vi "H_ofAllPoints.vi"(10 "Temperature Sensors":T2, 11 "Pressure Sensors in":T1) -> (3 "H's":dbl[](array[numeric]))   [LabVIEW 2017]
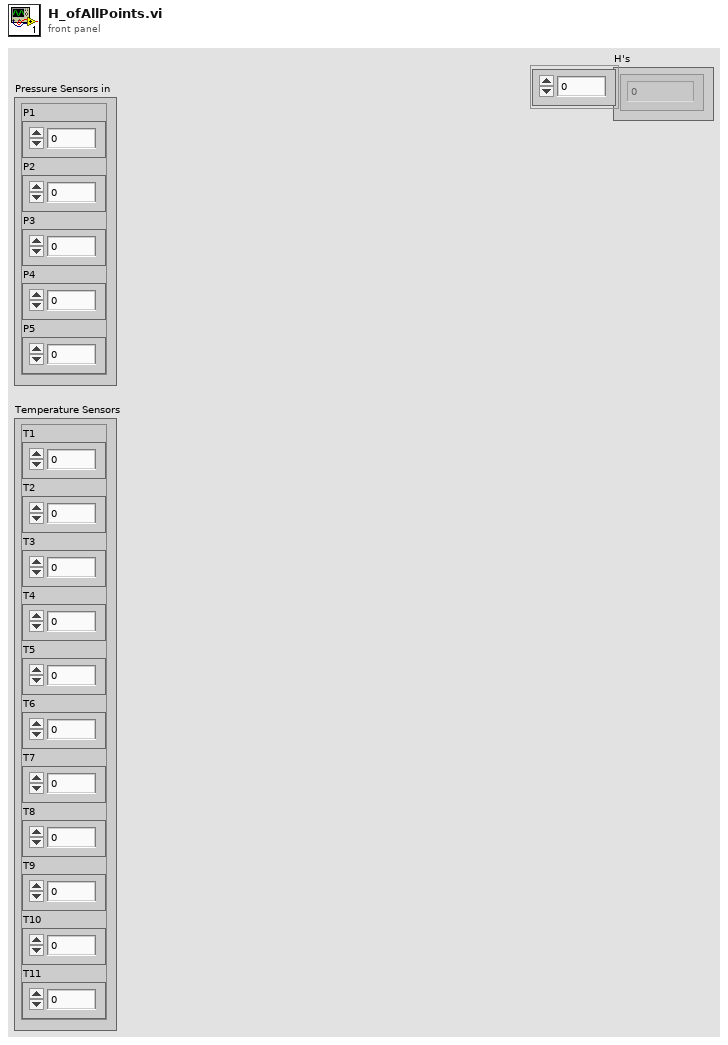
[diagram p1: front panel]
types:
  T1 = cluster{"P1":dbl, "P2":dbl, "P3":dbl, "P4":dbl, "P5":dbl}
  T2 = cluster{"T1":dbl, "T2":dbl, "T3":dbl, "T4":dbl, "T5":dbl, "T6":dbl, "T7":dbl, "T8":dbl, "T9":dbl, "T10":dbl, "T11":dbl}
  T3 = cluster{"S":dbl, "H":dbl, "V":dbl, "T":dbl, "P":dbl, "Status":enum16{"Sub Cooled", "Saturation", "Super Heated"}, "S 2":dbl, "H 2":dbl, "V 2":dbl, "T No":enum16{"0", "1", "2", "3", "4"}, "quality":dbl}
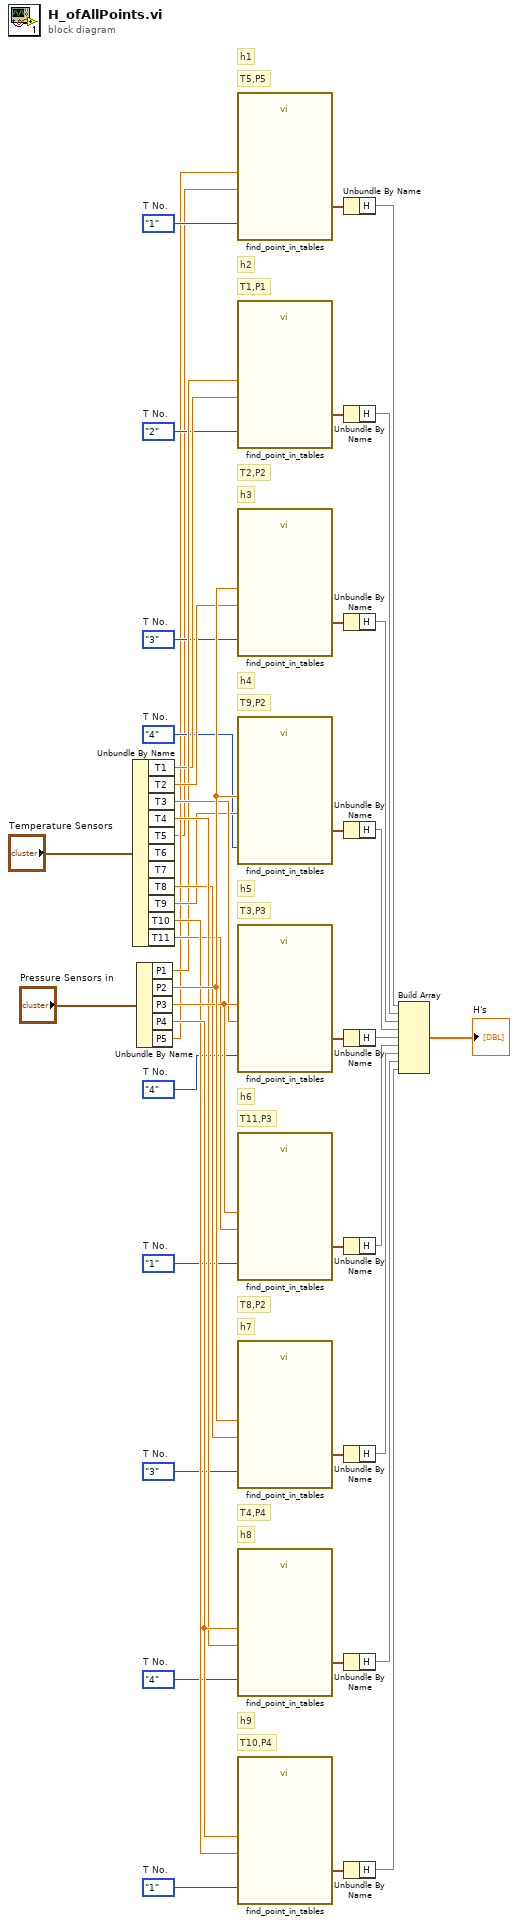
[diagram p0: block diagram]
diagram:
  w20 = enum16{"0", "1", "2", "3", "4"}."1"  # T No.
  w19 = enum16{"0", "1", "2", "3", "4"}."4"  # T No.
  w16 = enum16{"0", "1", "2", "3", "4"}."3"  # T No.
  w15 = enum16{"0", "1", "2", "3", "4"}."1"  # T No.
  w12 = enum16{"0", "1", "2", "3", "4"}."4"  # T No.
  w11 = enum16{"0", "1", "2", "3", "4"}."4"  # T No.
  w8 = enum16{"0", "1", "2", "3", "4"}."3"  # T No.
  w7 = enum16{"0", "1", "2", "3", "4"}."2"  # T No.
  w4 = enum16{"0", "1", "2", "3", "4"}."1"  # T No.
  # "T10,P4"
  # "T4,P4"
  # "T8,P2"
  # "T11,P3"
  # "T3,P3"
  # "T9,P2"
  # "T2,P2"
  # "T1,P1"
  # "T5,P5"
  # "h9"
  # "h8"
  # "h7"
  # "h6"
  # "h5"
  # "h4"
  # "h3"
  # "h2"
  # "h1"
  n1 = Unbundle By Name("Temperature Sensors") -> ("T1"=w22:dbl, "T2"=w24:dbl, "T3"=w26:dbl, "T4"=w29:dbl, "T5"=w2:dbl, "T8"=w28:dbl, "T9"=w25:dbl, "T10"=w30:dbl, "T11"=w27:dbl)  [unwired: 2 out]
  n2 = Unbundle By Name("Pressure Sensors in") -> ("P1"=w23:dbl, "P2"=w32:dbl, "P3"=w31:dbl, "P4"=w33:dbl, "P5"=w3:dbl)
  n3 = call "find_point_in_tables.vi"("T No."=w4, "T Search"=w2, "P Search"=w3) -> ("Point"=w5:T3)  [unwired: 7 in]
  n4 = call "find_point_in_tables.vi"("T No."=w7, "T Search"=w22, "P Search"=w23) -> ("Point"=w6:T3)  [unwired: 7 in]
  n5 = call "find_point_in_tables.vi"("T No."=w8, "T Search"=w24, "P Search"=w32) -> ("Point"=w9:T3)  [unwired: 7 in]
  n6 = call "find_point_in_tables.vi"("T No."=w11, "T Search"=w25, "P Search"=w32) -> ("Point"=w10:T3)  [unwired: 7 in]
  n7 = call "find_point_in_tables.vi"("T No."=w12, "T Search"=w26, "P Search"=w31) -> ("Point"=w13:T3)  [unwired: 7 in]
  n8 = call "find_point_in_tables.vi"("T No."=w15, "T Search"=w27, "P Search"=w31) -> ("Point"=w14:T3)  [unwired: 7 in]
  n9 = call "find_point_in_tables.vi"("T No."=w16, "T Search"=w28, "P Search"=w32) -> ("Point"=w17:T3)  [unwired: 7 in]
  n10 = call "find_point_in_tables.vi"("T No."=w19, "T Search"=w29, "P Search"=w33) -> ("Point"=w18:T3)  [unwired: 7 in]
  n11 = call "find_point_in_tables.vi"("T No."=w20, "T Search"=w30, "P Search"=w33) -> ("Point"=w21:T3)  [unwired: 7 in]
  n12 = Unbundle By Name(w5) -> ("H"=w34:dbl)
  n13 = Unbundle By Name(w6) -> ("H"=w35:dbl)
  n14 = Unbundle By Name(w9) -> ("H"=w36:dbl)
  n15 = Unbundle By Name(w10) -> ("H"=w37:dbl)
  n16 = Unbundle By Name(w13) -> ("H"=w38:dbl)
  n17 = Unbundle By Name(w14) -> ("H"=w39:dbl)
  n18 = Unbundle By Name(w17) -> ("H"=w40:dbl)
  n19 = Unbundle By Name(w18) -> ("H"=w41:dbl)
  n20 = Unbundle By Name(w21) -> ("H"=w42:dbl)
  n21 = Build Array(w34, w35, w36, w37, w38, w39, w40, w41, w42) -> (→"H's":dbl[])
